vi "EDVR.vi"() -> ()   [LabVIEW 2017]
panel:
  out "data value 2":dbl[][](array[numeric])
  out "data value":dbl[][](array[numeric])
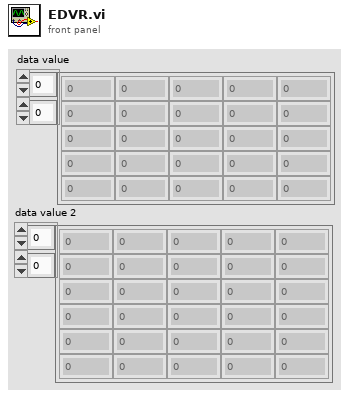
[diagram p1: front panel]
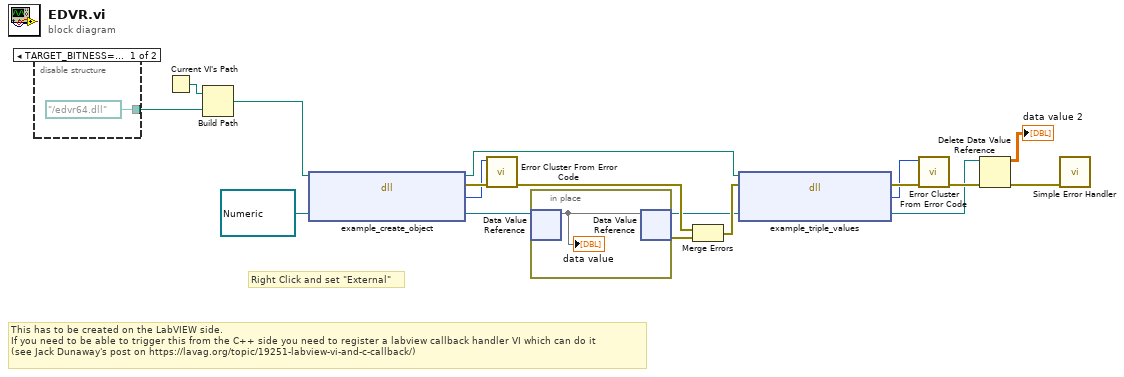
[diagram p0: block diagram]
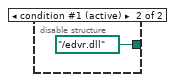
[diagram p2: hidden frame]
diagram:
  # "This has to be created on the LabVIEW side. \nIf you need to be able to trigger this from the C++ side you need to register a labview callback handler VI which can do it\n(see Jack Dunaway's post on https://lavag.org/topic/19251-labview-vi-and-c-callback/)"
  # "Right Click and set \"External\""
  n1 = disable-structure shown="TARGET_BITNESS==64" {
    disable-tunnel: [path "../edvr64.dll" ("name or relative path") path "../edvr.dll" ("name or relative path")] -> w1
    frame condition #0 {
    }
    frame condition #1 (active) {
    }
  }
  n2 = Current VI's Path() -> (path=w2:path)
  n3 = Build Path(base path=w2, name or relative path=w1) -> (appended path=w3:path)
  n4 = dll-call lib="?" fn="example_create_object"(path in=w3, "EDVR_Ref"=refnum<data-value> refnum ("data value reference")) -> (path out=w4:path, error out=w16:errorcluster, "Err"=w15:i32, "EDVR_Ref"=w14:refnum<data-value>)  [unwired: 2 in]
  n5 = call <vilib>:"Error Cluster From Error Code.vi"("error in (no error)"=w16, "error code (0)"=w15) -> ("error out"=w12:errorcluster)  [unwired: 7 in]
  n6 = in-place {
    n7 = in-place-dvr #1(w14) -> (w21:dbl[][])  [unwired: 1 out]
    "data value" <- w21
    n8 = in-place-dvr #1(w21) -> (w10:refnum<data-value>, w13:errorcluster)
  }
  n9 = Merge Errors(w12, w13) -> (w11:errorcluster)
  n10 = dll-call lib="?" fn="example_triple_values"(path in=w4, error in=w11, "EDVR_Ref"=w10) -> (error out=w9:errorcluster, "Err"=w8:i32, "EDVR_Ref"=w7:refnum<data-value>)  [unwired: 1 in, 1 out]
  n11 = call <vilib>:"Error Cluster From Error Code.vi"("error in (no error)"=w9, "error code (0)"=w8) -> ("error out"=w18:errorcluster)  [unwired: 7 in]
  n12 = Delete Data Value Reference(data value reference=w7, error in=w18) -> (data value=→"data value 2":dbl[][], error out=w5:errorcluster)
  n13 = call <vilib>:"Simple Error Handler.vi"("error in (no error)"=w5) -> ()  [unwired: 4 in, 5 out]
